vi "Get Intermediate Result.vi"(11 "error in (no error)":errorcluster) -> (4 "Intermediate Result":T1[](array[typedef]), 15 "error out":errorcluster)   [LabVIEW 2023, in "RFFixtureCharact.Public.lvlib" / "Vector Abstract Path.lvclass"]
uses:
  Vector Abstract Path.lvclass
  Instruments/Cal Standard/Type Definitions/One-Port Charact Data.ctl
  Instruments/Cal Standard/Type Definitions/Standard Type.ctl
  Vector Abstract Path.lvclass/Vector Abstract Path.ctl
  RFFixtureCharact.Public.lvlib
  Instruments/RFFixtureCharact.Instruments.lvlib
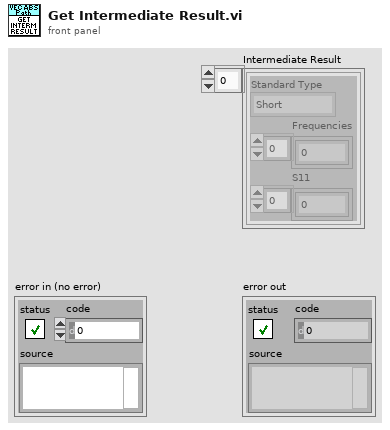
[diagram p1: front panel]
types:
  T1 = typedef "RFFixtureCharact.Instruments.lvlib/One-Port Charact Data.ctl" = cluster{"Standard Type":T2, "Frequencies":dbl[], "S11":cdb[]}
  T2 = typedef "RFFixtureCharact.Instruments.lvlib/Standard Type.ctl" = enum16{"Short", "Open", "Load", "PowerMeter", "None"}
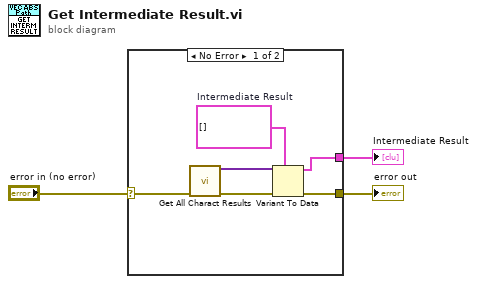
[diagram p0: block diagram]
diagram:
  n1 = case shown="No Error" "error in (no error)" {
    selector: "error in (no error)" -> [w5 w10]
    tunnel: [w8 w10] -> w2
    tunnel: [w7 _] -> w1
    frame No Error {
      w9 = T1[] []  # Intermediate Result
      n2 = call "Get All Charact Results.vi"("error in"=w5) -> ("All Cal Results"=w6:variant[], "error out"=w4:errorcluster)  [unwired: 13 in]
      n3 = Variant To Data(error in=w4, type=w9, Variant=w6) -> (data=w7:T1[], error out=w8:errorcluster)
    }
    frame Error {
    }
  }
  "error out" <- w2
  "Intermediate Result" <- w1
